vi "GetPaths.vi"() -> (1 "Libraries path":path, 3 "Templates path":path)   [LabVIEW 2016]
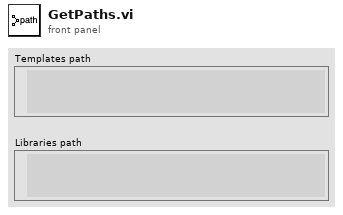
[diagram p1: front panel]
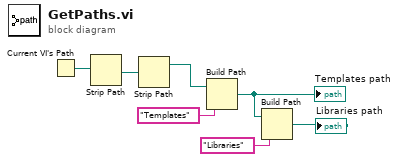
[diagram p0: block diagram]
diagram:
  n1 = Current VI's Path() -> (path=w5:path)
  n2 = Strip Path(path=w5) -> (stripped path=w6:path)  [unwired: 1 out]
  n3 = Strip Path(path=w6) -> (stripped path=w7:path)  [unwired: 1 out]
  n4 = Build Path(base path=w7, name or relative path="Templates") -> (appended path=w2:path)
  "Templates path" <- w2
  n5 = Build Path(base path=w2, name or relative path="Libraries") -> (appended path=→"Libraries path":path)
